vi "示波器_v1.0.vi"() -> ()   [LabVIEW 2014]
uses:
  <vilib>/Utility/file.llb/Write To Spreadsheet File (DBL).vi
panel:
  out "波形图":dbl[](graph)
  in  "刷新间隔/ms":u32=100
  out "写入深度显示":dbl
  in  "触发阈值":dbl
  out "示波器":bool
  out "是否触发":bool
  in  "文件路径输入控件":path
  in  "保存按钮":bool
  in  "停止":bool
  in  "开始":bool
  in  "触发次数":enum16{"单次触发", "连续触发"}(ring)
  in  "触发方式":enum16{"大于阈值触发", "小于阈值触发", "强制触发"}(ring)
  in  "X position":u16(knob) scale=0.0..8191.0
  in  "通讯":enum16{"空闲", "配置", "是否触发？", "读取波形数据"}(ring)
  in  "按键状态监测":enum16{"空闲", "开始", "停止", "保存", "退出"}(ring)
  # "示波器"
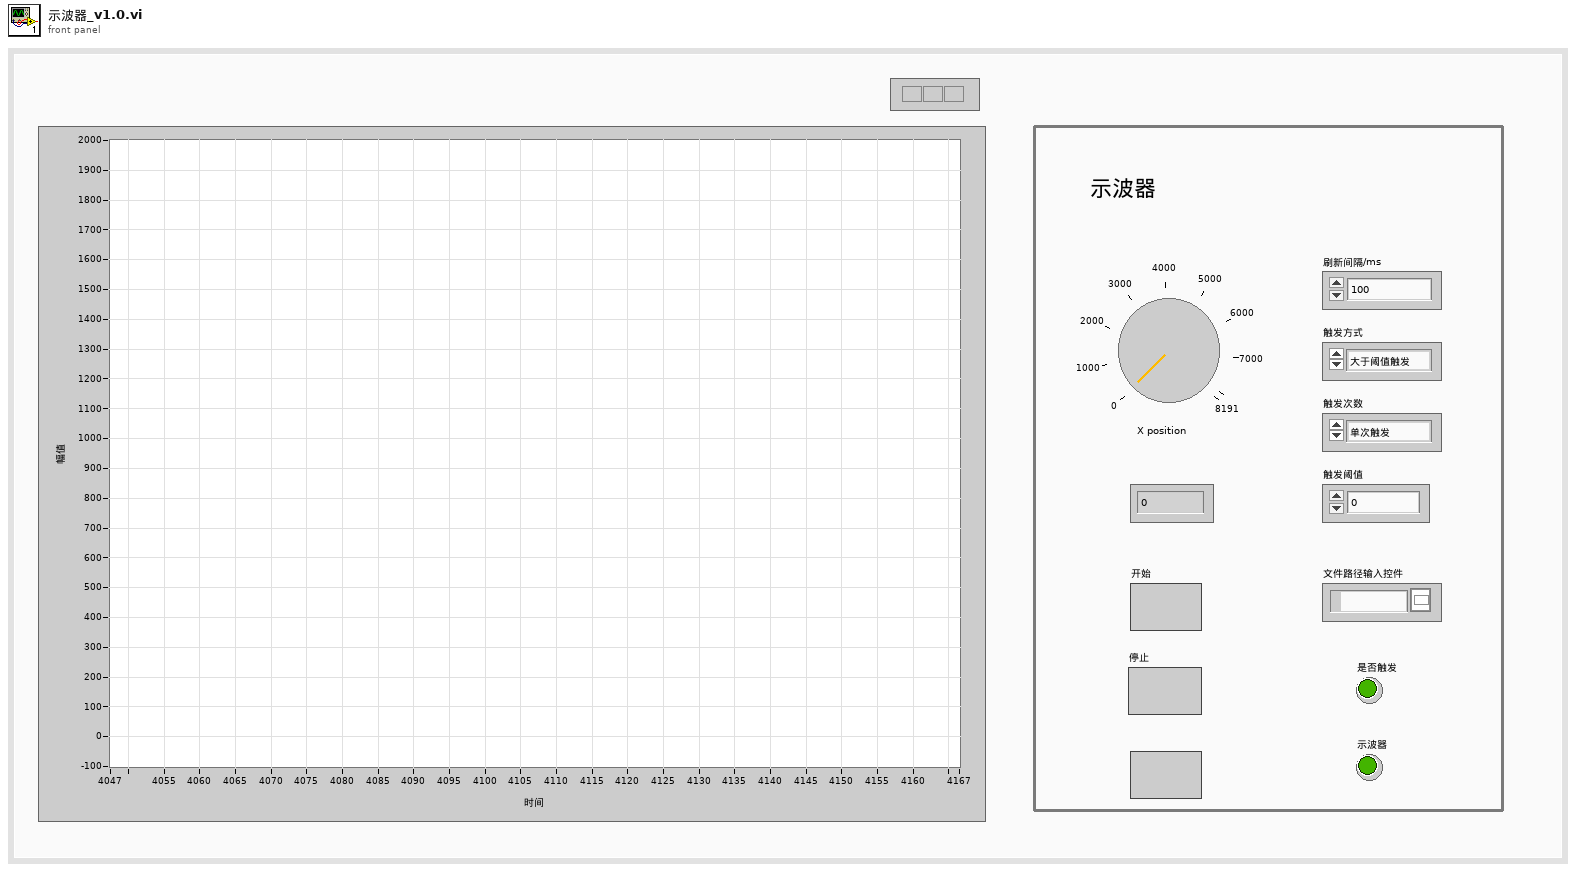
[diagram p1: front panel]
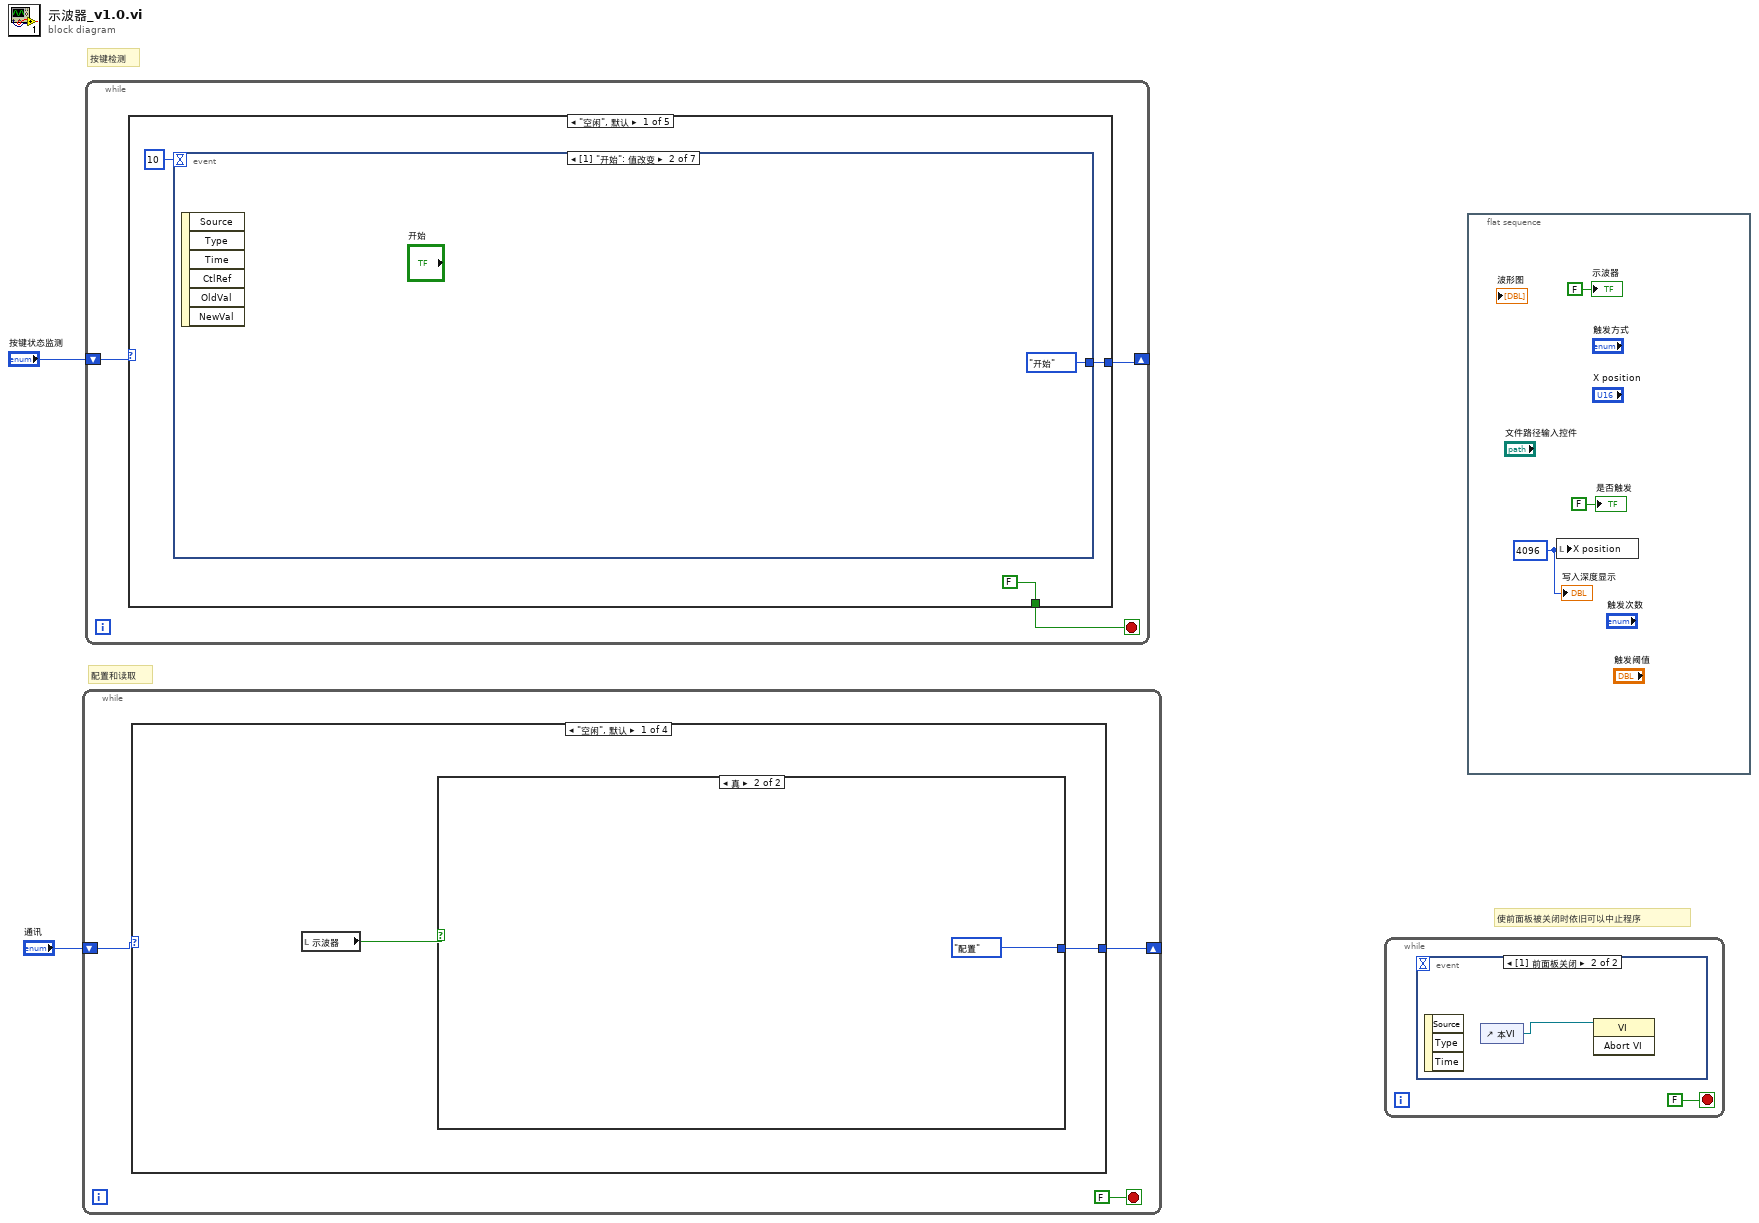
[diagram p0: block diagram]
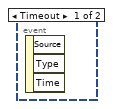
[diagram p2: hidden frame]
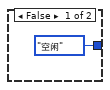
[diagram p3: hidden frame]
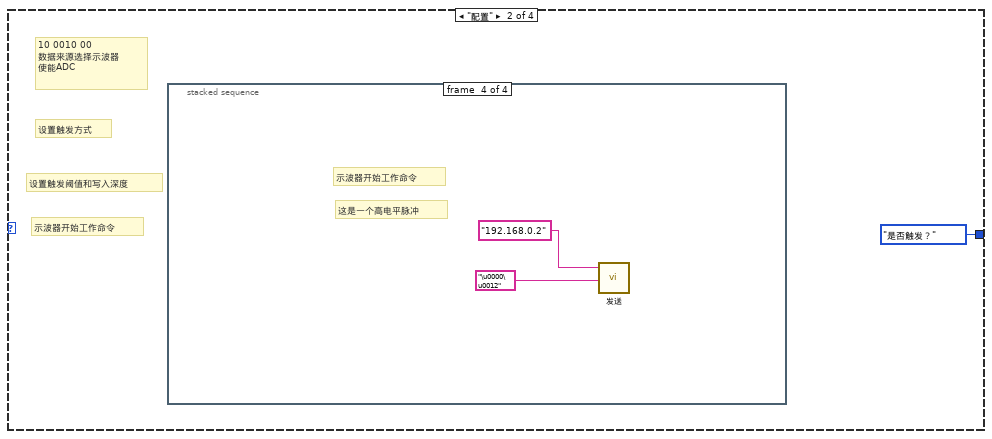
[diagram p4: hidden frame]
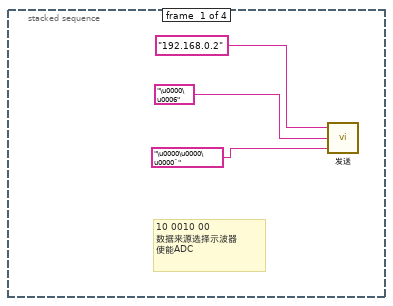
[diagram p5: hidden frame]
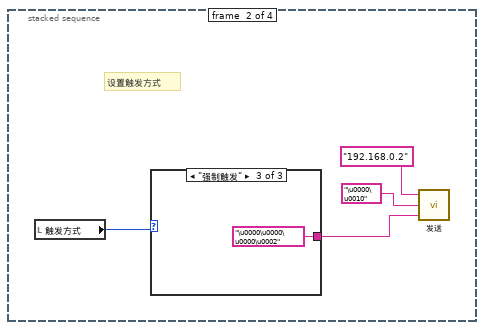
[diagram p6: hidden frame]
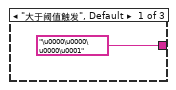
[diagram p7: hidden frame]
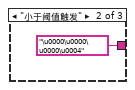
[diagram p8: hidden frame]
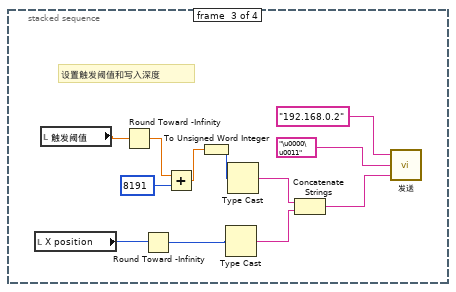
[diagram p9: hidden frame]
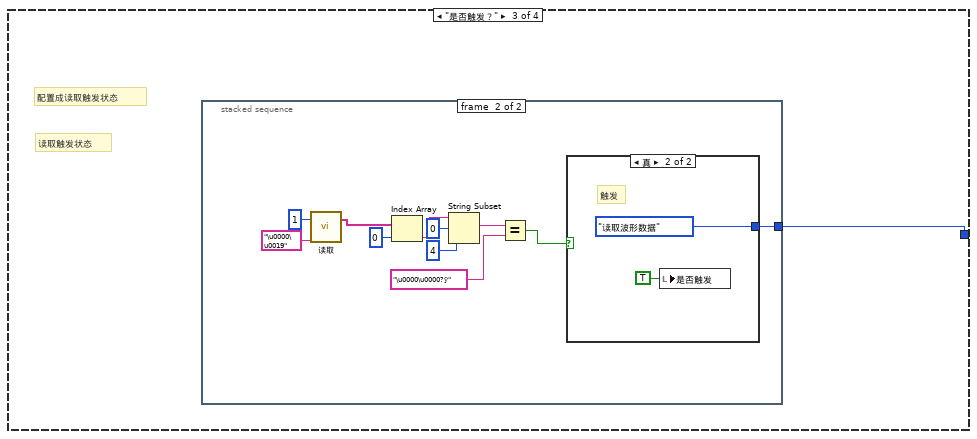
[diagram p10: hidden frame]
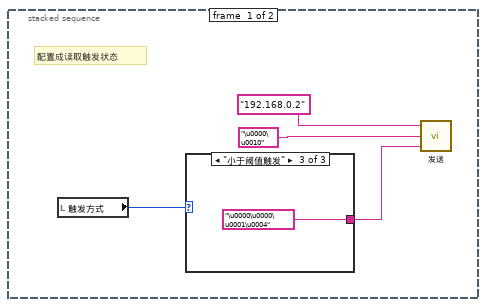
[diagram p11: hidden frame]
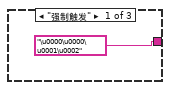
[diagram p12: hidden frame]
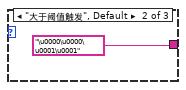
[diagram p13: hidden frame]
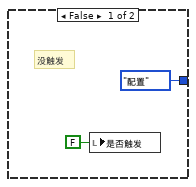
[diagram p14: hidden frame]
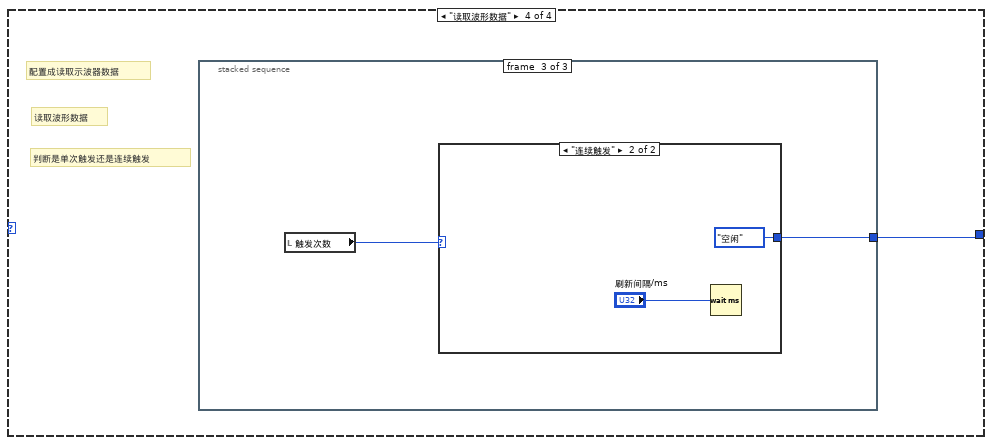
[diagram p15: hidden frame]
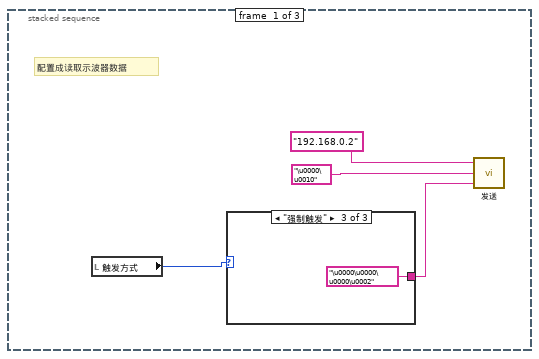
[diagram p16: hidden frame]
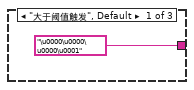
[diagram p17: hidden frame]
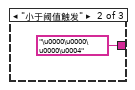
[diagram p18: hidden frame]
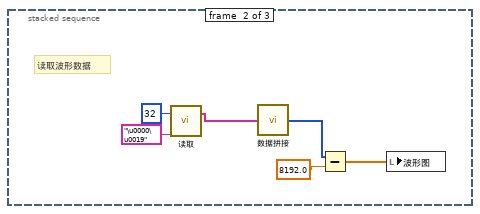
[diagram p19: hidden frame]
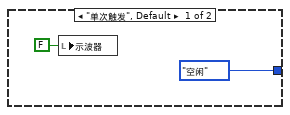
[diagram p20: hidden frame]
diagram:
  # "使前面板被关闭时依旧可以中止程序"
  # "配置和读取"
  # "按键检测"
  n1 = while {
    shift-right: [w3] -> _
    shift-left: "通讯" -> [w4]
    stop <- FALSE stop-if-true
    n2 = case shown="\"空闲\", 默认" w4 {
      tunnel: [w7 enum16{"空闲", "配置", "是否触发？", "读取波形数据"}."是否触发？" ("通讯") w35 w58] -> w3
      frame "空闲", Default {
        n3 = local read "示波器"() -> (w6:bool)
        n4 = case shown="真" w6 {
          tunnel: [enum16{"空闲", "配置", "是否触发？", "读取波形数据"}."空闲" ("通讯") enum16{"空闲", "配置", "是否触发？", "读取波形数据"}."配置" ("通讯")] -> w7
          frame False {
          }
          frame True {
          }
        }
      }
      frame "配置" {
        # "示波器开始工作命令"
        # "设置触发阈值和写入深度"
        # "设置触发方式"
        # "10 0010 00\n数据来源选择示波器\n使能ADC"
        n5 = stacked-sequence {
          frame #0 {
            # "10 0010 00\n数据来源选择示波器\n使能ADC"
            n6 = call "发送.vi"("数据（32bit）"="\u0000\u0000\u0000ˆ", "命令(16bit)"="\u0000\u0006", "目标IP"="192.168.0.2") -> ()  [unwired: 1 out]
          }
          frame #1 {
            # "设置触发方式"
            n7 = local read "触发方式"() -> (w15:enum16{"大于阈值触发", "小于阈值触发", "强制触发"})
            n8 = case shown="\"强制触发\"" w15 {
              tunnel: ["\u0000\u0000\u0000\u0001" "\u0000\u0000\u0000\u0004" "\u0000\u0000\u0000\u0002"] -> w14
              frame "大于阈值触发", Default {
              }
              frame "小于阈值触发" {
              }
              frame "强制触发" {
              }
            }
            n9 = call "发送.vi"("数据（32bit）"=w14, "命令(16bit)"="\u0000\u0010", "目标IP"="192.168.0.2") -> ()  [unwired: 1 out]
          }
          frame #2 {
            # "设置触发阈值和写入深度"
            n10 = local read "X position"() -> (w26:u16)
            n11 = local read "触发阈值"() -> (w24:dbl)
            n12 = Round Toward -Infinity(1:w24) -> (0:w23:dbl)
            n13 = Round Toward -Infinity(1:w26) -> (0:w25:u16)
            n14 = Add(x=w23, y=u16 8191) -> (x+y=w22:dbl)
            n15 = To Unsigned Word Integer(number=w22) -> (unsigned 16bit integer=w21:u16)
            n16 = Type Cast(x=w25) -> (*(type *) &x=w29:string)  [unwired: 1 in]
            n17 = Type Cast(x=w21) -> (*(type *) &x=w30:string)  [unwired: 1 in]
            n18 = Concatenate Strings(w30, w29) -> (w28:string)
            n19 = call "发送.vi"("数据（32bit）"=w28, "命令(16bit)"="\u0000\u0011", "目标IP"="192.168.0.2") -> ()  [unwired: 1 out]
          }
          frame #3 {
            # "这是一个高电平脉冲"
            # "示波器开始工作命令"
            n20 = call "发送.vi"("命令(16bit)"="\u0000\u0012", "目标IP"="192.168.0.2") -> ()  [unwired: 1 in, 1 out]
          }
        }
      }
      frame "是否触发？" {
        # "读取触发状态"
        # "配置成读取触发状态"
        n21 = stacked-sequence {
          tunnel: [_ w43] -> w35
          frame #0 {
            # "配置成读取触发状态"
            n22 = local read "触发方式"() -> (w37:enum16{"大于阈值触发", "小于阈值触发", "强制触发"})
            n23 = case shown="\"小于阈值触发\"" w37 {
              tunnel: ["\u0000\u0000\u0001\u0002" ("数据（32bit）") "\u0000\u0000\u0001\u0001" ("数据（32bit）") "\u0000\u0000\u0001\u0004" ("数据（32bit）")] -> w36
              frame "强制触发" {
              }
              frame "大于阈值触发", Default {
              }
              frame "小于阈值触发" {
              }
            }
            n24 = call "发送.vi"("数据（32bit）"=w36, "命令(16bit)"="\u0000\u0010", "目标IP"="192.168.0.2") -> ()  [unwired: 1 out]
          }
          frame #1 {
            n25 = call "读取.vi"("命令"="\u0000\u0019", "帧数"=1) -> ("数组"=w51:string[])  [unwired: 1 out]
            n26 = Index Array(array=w51, index=0 ("索引")) -> (element=w49:string)
            n27 = String Subset(string=w49, offset (0)=0 ("偏移量(0)"), length (rest)=4 ("长度（剩余）")) -> (substring=w46:string)
            n28 = Equal?(x=w46, y="\u0000\u0000?ÿ") -> (x = y?=w44:bool)
            n29 = case shown="真" w44 {
              tunnel: [enum16{"空闲", "配置", "是否触发？", "读取波形数据"}."配置" ("通讯") enum16{"空闲", "配置", "是否触发？", "读取波形数据"}."读取波形数据" ("通讯")] -> w43
              frame False {
                # "没触发"
                n30 = local write "是否触发"(FALSE ("是否触发")) -> ()
              }
              frame True {
                # "触发"
                n31 = local write "是否触发"(TRUE ("是否触发")) -> ()
              }
            }
          }
        }
      }
      frame "读取波形数据" {
        # "判断是单次触发还是连续触发"
        # "读取波形数据"
        # "配置成读取示波器数据"
        n32 = stacked-sequence {
          tunnel: [_ _ w72] -> w58
          frame #0 {
            # "配置成读取示波器数据"
            n33 = local read "触发方式"() -> (w60:enum16{"大于阈值触发", "小于阈值触发", "强制触发"})
            n34 = case shown="\"强制触发\"" w60 {
              tunnel: ["\u0000\u0000\u0000\u0001" ("数据（32bit）") "\u0000\u0000\u0000\u0004" ("数据（32bit）") "\u0000\u0000\u0000\u0002" ("数据（32bit）")] -> w59
              frame "大于阈值触发", Default {
              }
              frame "小于阈值触发" {
              }
              frame "强制触发" {
              }
            }
            n35 = call "发送.vi"("数据（32bit）"=w59, "命令(16bit)"="\u0000\u0010", "目标IP"="192.168.0.2") -> ()  [unwired: 1 out]
          }
          frame #1 {
            # "读取波形数据"
            n36 = call "读取.vi"("命令"="\u0000\u0019", "帧数"=32) -> ("数组"=w69:string[])  [unwired: 1 out]
            n37 = call "数据拼接.vi"("数组"=w69) -> ("输出数据"=w68:i32[])
            n38 = Subtract(x=w68, y=8192.0) -> (x-y=w66:dbl[])
            n39 = local write "波形图"(w66) -> ()
          }
          frame #2 {
            n40 = local read "触发次数"() -> (w73:enum16{"单次触发", "连续触发"})
            n41 = case shown="\"连续触发\"" w73 {
              tunnel: [enum16{"空闲", "配置", "是否触发？", "读取波形数据"}."空闲" ("通讯") enum16{"空闲", "配置", "是否触发？", "读取波形数据"}."空闲" ("通讯")] -> w72
              frame "单次触发", Default {
                n42 = local write "示波器"(FALSE ("示波器")) -> ()
              }
              frame "连续触发" {
                n43 = Wait (ms)(milliseconds to wait="刷新间隔/ms") -> ()  [unwired: 1 out]
              }
            }
          }
        }
      }
    }
  }
  n44 = while {
    shift-right: [w79] -> _
    shift-left: "按键状态监测" -> [w80]
    stop <- w78 stop-if-true
    n45 = case shown="\"空闲\", 默认" w80 {
      tunnel: [w82 enum16{"空闲", "开始", "停止", "保存", "退出"}."空闲" ("按键状态监测") enum16{"空闲", "开始", "停止", "保存", "退出"}."空闲" ("按键状态监测") enum16{"空闲", "开始", "停止", "保存", "退出"}."空闲" ("按键状态监测") enum16{"空闲", "开始", "停止", "保存", "退出"}."空闲" ("按键状态监测")] -> w79
      tunnel: [FALSE FALSE FALSE FALSE TRUE] -> w78
      frame "空闲", Default {
        n46 = event shown="[1] \"开始\": 值改变" {
          selector: _ -> [_ _ _ _ _ _ _]
          dyn-events: _ -> [_ _ _ _ _ _ _]
          timeout: 10 -> [_ _ _ _ _ _ _]
          tunnel: [enum16{"空闲", "开始", "停止", "保存", "退出"}."空闲" ("按键状态监测") enum16{"空闲", "开始", "停止", "保存", "退出"}."开始" ("按键状态监测") enum16{"空闲", "开始", "停止", "保存", "退出"}."停止" ("按键状态监测") _ _ enum16{"空闲", "开始", "停止", "保存", "退出"}."空闲" ("按键状态监测") enum16{"空闲", "开始", "停止", "保存", "退出"}."保存" ("按键状态监测")] -> w82
          event Timeout {
            n47 = event-data() -> ()  [unwired: 1 in, 3 out]
          }
          event "开始": Value Change {
            n48 = event-data() -> ()  [unwired: 1 in, 6 out]
          }
          event "停止": Value Change {
            n49 = event-data() -> ()  [unwired: 1 in, 6 out]
          }
          event "波形图": Cursor Move {
            n50 = event-data() -> ()  [unwired: 1 in, 9 out]
            n51 = property on="波形图" class="WFGraph (严格)"() -> ("Cursor.Cursor Y"=w87:dbl)  [unwired: 2 in, 2 out]
            n52 = Round Toward -Infinity(1:w87) -> (0:w88:dbl)
            n53 = local write "触发阈值"(w88) -> ()
          }
          event "触发阈值": Value Change {
            n54 = event-data() -> ()  [unwired: 1 in, 6 out]
            n55 = local read "触发阈值"() -> (w90:dbl)
            n56 = Round Toward -Infinity(1:w90) -> (0:w89:dbl)
            n57 = property on="波形图" class="WFGraph (严格)"("Cursor.Cursor Y"=w89) -> ()  [unwired: 2 in, 2 out]
          }
          event "X position": Value Change {
            n58 = event-data() -> ()  [unwired: 1 in, 6 out]
            n59 = local read "X position"() -> (w93:u16)
            n60 = Round Toward -Infinity(1:w93) -> (0:w92:u16)
            n61 = local write "写入深度显示"(w92) -> ()
          }
          event "保存按钮": Value Change {
            n62 = event-data() -> ()  [unwired: 1 in, 6 out]
          }
        }
      }
      frame "开始" {
        n63 = local write "示波器"(TRUE ("示波器")) -> ()
      }
      frame "停止" {
        n64 = local write "示波器"(FALSE ("示波器")) -> ()
      }
      frame "保存" {
        n65 = local read "文件路径输入控件"() -> (w101:path)
        n66 = Equal?(x=w101, y=path "") -> (x = y?=w103:bool)
        n67 = case shown="假" w103 {
          tunnel: w101 -> [w109 _]
          frame False {
            n68 = local read "波形图"() -> (w108:dbl[])
            n69 = call-poly <vilib>:"Write To Spreadsheet File.vi"("transpose? (no:F)"=TRUE, "1D data"=w108, "file path (dialog if empty)"=w109) -> ()  [unwired: 5 in, 1 out]
            n70 = One Button Dialog(message="保存成功" ("消息")) -> ()  [unwired: 1 in, 1 out]
          }
          frame True {
            n71 = One Button Dialog(message="请输入存储路径" ("消息")) -> ()  [unwired: 1 in, 1 out]
          }
        }
      }
      frame "退出" {
      }
    }
  }
  n72 = while {
    stop <- FALSE stop-if-true
    n73 = event shown="[1] 前面板关闭" {
      selector: _ -> [_ _]
      dyn-events: _ -> [_ _]
      timeout: _ -> [_ _]
      event Timeout {
        n74 = event-data() -> ()  [unwired: 1 in, 3 out]
      }
      event Panel Close {
        n75 = event-data() -> ()  [unwired: 1 in, 3 out]
        n76 = control-ref of="本VI"() -> (w114:refnum<vi>)
        n77 = invoke class="VI" method="Abort VI"(reference=w114) -> ()  [unwired: 2 in, 3 out]
      }
    }
  }
  n78 = flat-sequence {
    frame #0 {
      w115 = u16 4096 ("X position")
      n79 = local write "X position"(w115) -> ()
      "是否触发" <- FALSE ("是否触发")
      "示波器" <- FALSE ("示波器")
      "写入深度显示" <- w115
    }
  }
